vi "Teleop.vi"(10 "Match Info":T1={"Autonomous Elapsed Seconds"=0.0, "TeleOp Elapsed Seconds"=0.0, "Disabled Elapsed Seconds"=0.0, "Visited Autonomous"=FALSE, "Visited TeleOp"=FALSE, "Visited Disabled"=FALSE, "Autonomous Settings"={"Autonomous Style"=enum."Independent", "VI Refnum"=refnum}}, 11 "Call Context":T2) -> ()   [LabVIEW 2012]
doc: "This VI is called for each TeleOp packet received from the DS where the robot is not disabled. It is often used to read from the joysticks and update I/O or to update setpoints for timed control loops. It should complete and return within 20 milliseconds or it may miss DS packets."
uses:
  <vilib>/Rock Robotics/WPI/DriverStation/WPI_DriverStationDerivedRobotMode.ctl
  <vilib>/Rock Robotics/WPI/DriverStation/WPI_DriverStationMatch Info.ctl
  Robot Global Data.vi
  <vilib>/Rock Robotics/WPI/Solenoid/Deprecated/WPI_SolenoidSetBool.vi
  <vilib>/Rock Robotics/WPI/Joystick/WPI_JoystickGetSetRefNum.vi
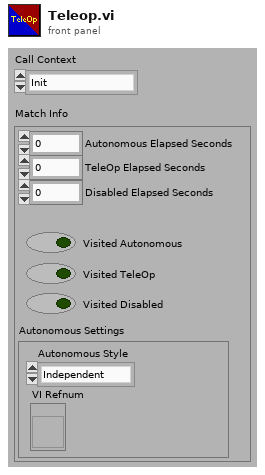
[diagram p1: front panel]
types:
  T1 = typedef "WPI_DriverStationMatch Info.ctl" = cluster{"Autonomous Elapsed Seconds":dbl, "TeleOp Elapsed Seconds":dbl, "Disabled Elapsed Seconds":dbl, "Visited Autonomous":bool, "Visited TeleOp":bool, "Visited Disabled":bool, "Autonomous Settings":cluster{"Autonomous Style":enum16{"Iterative", "Independent"}, "VI Refnum":refnum<vi>}}
  T2 = typedef "WPI_DriverStationDerivedRobotMode.ctl" = enum16{"Init", "Execute", "Stop"}
  T3 = typedef "WPI_DigitalInputDevRef.ctl" = cluster{"DevStatus":errorcluster, "DIO Channel":T4, "Digital Module":T5}
  T4 = typedef "FPGA_DIOChannel.ctl" = enum8{"DIO 1", "DIO 2", "DIO 3", "DIO 4", "DIO 5", "DIO 6", "DIO 7", "DIO 8", "DIO 9", "DIO 10", "DIO 11", "DIO 12", "DIO 13", "DIO 14", "Invalid"}
  T5 = typedef "FPGA_TypedefDigitalModule.ctl" = enum16{"Digital Module 1", "Digital Module 2"}
  T6 = typedef "WPI_SolenoidDevRef.ctl" = cluster{"DevStatus":errorcluster, "Solenoid Module":T7, "Forward Solenoid Channel":T8, "Reverse Solenoid Channel":T8}
  T7 = typedef "FPGA_TypedefSolenoidModule.ctl" = enum16{"Solenoid Module 1", "Solenoid Module 2"}
  T8 = typedef "WPI_SolenoidChannel.ctl" = enum8{"Solenoid 1", "Solenoid 2", "Solenoid 3", "Solenoid 4", "Solenoid 5", "Solenoid 6", "Solenoid 7", "Solenoid 8", "Invalid"}
  T9 = typedef "WPI_MotorControlDeviceRef.ctl" = cluster{"DeviceStatus":errorcluster, "Type":enum16{"PWM", "CAN"}, "PWM":cluster{"Digital Module":T5, "PWM Channel":T10, "DeadBand":T11}, "CAN":cluster{"Device Number":u8, "Control Mode":T12, "Semaphore":T13, "Max Vout":dbl}, "Invert":bool, "TransformRef":T14, "InvTransformRef":T14}
  T10 = typedef "FPGA_DIOPWMChannel.ctl" = enum8{"PWM 1", "PWM 2", "PWM 3", "PWM 4", "PWM 5", "PWM 6", "PWM 7", "PWM 8", "PWM 9", "PWM 10", "Invalid"}
  T11 = typedef "WPI_PWMDeadband.ctl" = cluster{"Name":string, "maxPositivePwm":i32, "minPositivePwm":i32, "centerPwm":i32, "maxNegativePwm":i32, "minNegativePwm":i32, "angularRange":u16}
  T12 = typedef "WPI_CANJaguar_ControlMode.ctl" = enum8{"Percent VBus", "Current", "Speed", "Position", "Voltage"}
  T13 = typedef "Semaphore RefNum" = refnum<k1>
  T14 = typedef "WPI_PWMTransform_ConPane.ctl" = refnum<vi>
  T15 = typedef "WPI_JoystickDevRef.ctl" = cluster{"Device":T16}
  T16 = typedef "WPI_JoystickDeviceEnum.ctl" = enum16{"USB 1", "USB 2", "USB 3", "USB 4", "Kinect 1", "Kinect 2"}
  T17 = typedef "WPI_JoystickButtonState.ctl" = cluster{"Button 1":bool, "Button 2":bool, "Button 3":bool, "Button 4":bool, "Button 5":bool, "Button 6":bool, "Button 7":bool, "Button 8":bool, "Button 9":bool, "Button 10":bool, "Button 11":bool, "Button 12":bool}
  T18 = cluster{"axis 1 (x)":dbl, "axis 2 (y)":dbl, "axis 3 (throttle)":dbl, "axis 4":dbl, "axis 5":dbl, "axis 6":dbl}
  T19 = typedef "WPI_RobotDriveDevRef.ctl" = cluster{"DevStatus":errorcluster, "Motors[]":T9[], "Square Inputs":bool, "Max Output":dbl, "Isochronous":bool}
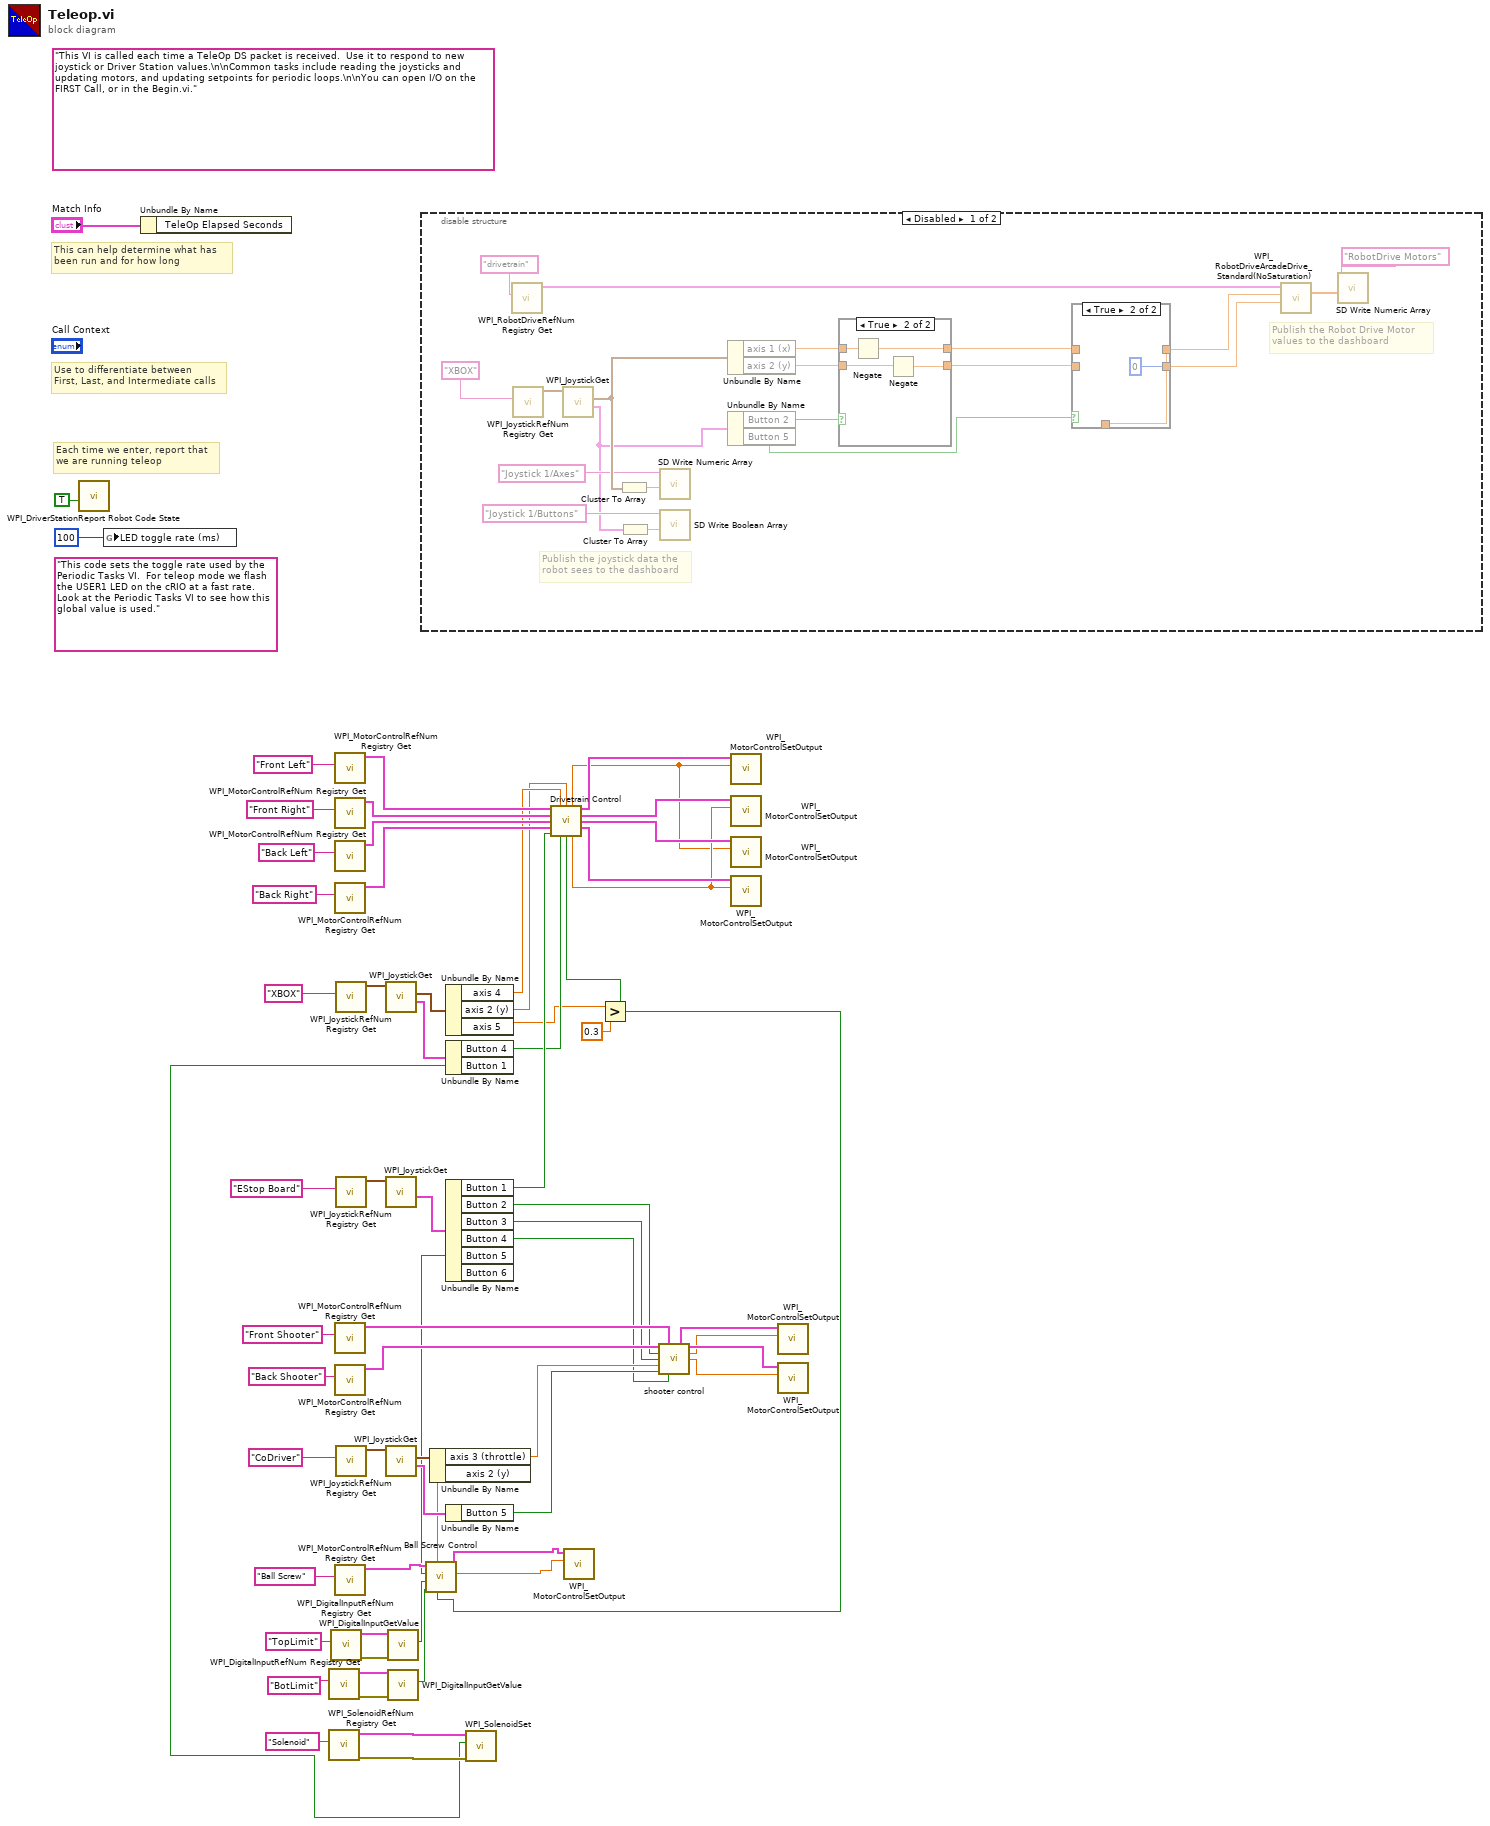
[diagram p0: block diagram]
diagram:
  (unwired) "This code sets the toggle rate used by the Periodic Tasks VI.  For teleop mode we flash the USER1 LED on the cRIO at a fast rate.  Look at the Periodic Tasks VI to see how this global value is used."
  (unwired) "This VI is called each time a TeleOp DS packet is received.  Use it to respond to new joystick or Driver Station values.\n\nCommon tasks include reading the joysticks and updating motors, and updating setpoints for periodic loops.\n\nYou can open I/O on the FIRST Call, or in the Begin.vi."
  # "Each time we enter, report that\nwe are running teleop"
  # "Use to differentiate between\nFirst, Last, and Intermediate calls"
  # "This can help determine what has\nbeen run and for how long"
  n1 = call <vilib>:"WPI_DriverStationReport Robot Code State.vi"("TeleOp"=TRUE ("Autonomous")) -> ()  [unwired: 10 in, 1 out]
  n2 = global write "Robot Global Data.vi" "LED toggle rate (ms)"(u32 100 ("LED ms toggle rate")) -> ()
  n3 = Unbundle By Name("Match Info") -> ()  [unwired: 1 out]
  n4 = call <vilib>:"WPI_DigitalInputRefNum Registry Get.vi"("refnum name"="BotLimit") -> ("error out"=w14:errorcluster, "DigitalInputDevRef"=w13:T3)  [unwired: 9 in]
  n5 = call <vilib>:"WPI_SolenoidRefNum Registry Get.vi"("refnum name"="Solenoid") -> ("error out"=w2:errorcluster, "SolenoidDevRef"=w3:T6)  [unwired: 9 in]
  n6 = call <vilib>:"WPI_DigitalInputRefNum Registry Get.vi"("refnum name"="TopLimit") -> ("error out"=w16:errorcluster, "DigitalInputDevRef"=w15:T3)  [unwired: 9 in]
  n7 = call <vilib>:"WPI_MotorControlRefNum Registry Get.vi"("refnum name"="Front Left") -> ("MotorControlDevRef"=w56:T9)  [unwired: 9 in, 1 out]
  n8 = call <vilib>:"WPI_MotorControlRefNum Registry Get.vi"("refnum name"="Front Right") -> ("MotorControlDevRef"=w55:T9)  [unwired: 9 in, 1 out]
  n9 = call <vilib>:"WPI_MotorControlRefNum Registry Get.vi"("refnum name"="Back Left") -> ("MotorControlDevRef"=w54:T9)  [unwired: 9 in, 1 out]
  n10 = call <vilib>:"WPI_MotorControlRefNum Registry Get.vi"("refnum name"="Back Right") -> ("MotorControlDevRef"=w53:T9)  [unwired: 9 in, 1 out]
  n11 = call <vilib>:"WPI_MotorControlRefNum Registry Get.vi"("refnum name"="Front Shooter") -> ("MotorControlDevRef"=w31:T9)  [unwired: 9 in, 1 out]
  n12 = call <vilib>:"WPI_MotorControlRefNum Registry Get.vi"("refnum name"="Back Shooter") -> ("MotorControlDevRef"=w32:T9)  [unwired: 9 in, 1 out]
  n13 = call <vilib>:"WPI_MotorControlRefNum Registry Get.vi"("refnum name"="Ball Screw") -> ("MotorControlDevRef"=w18:T9)  [unwired: 9 in, 1 out]
  n14 = call <vilib>:"WPI_JoystickRefNum Registry Get.vi"("refnum name"="XBOX") -> ("JoystickDevRef"=w51:T15)  [unwired: 1 in, 9 out]
  n15 = call <vilib>:"WPI_JoystickRefNum Registry Get.vi"("refnum name"="EStop Board") -> ("JoystickDevRef"=w41:T15)  [unwired: 1 in, 9 out]
  n16 = call <vilib>:"WPI_JoystickRefNum Registry Get.vi"("refnum name"="CoDriver") -> ("JoystickDevRef"=w45:T15)  [unwired: 1 in, 9 out]
  n17 = call <vilib>:"WPI_JoystickGet.vi"("JoystickDevRef"=w51) -> ("Buttons"=w47:T17, "Axes"=w50:T18)  [unwired: 1 in, 4 out]
  n18 = call <vilib>:"WPI_JoystickGet.vi"("JoystickDevRef"=w41) -> ("Buttons"=w40:T17)  [unwired: 1 in, 5 out]
  n19 = call <vilib>:"WPI_JoystickGet.vi"("JoystickDevRef"=w45) -> ("Buttons"=w43:T17, "Axes"=w44:T18)  [unwired: 1 in, 4 out]
  n20 = call <vilib>:"WPI_DigitalInputGetValue.vi"("error in (no error)"=w16, "DigitalInputDevRef"=w15) -> ("Value"=w12:bool)  [unwired: 7 in, 2 out]
  n21 = call <vilib>:"WPI_DigitalInputGetValue.vi"("error in (no error)"=w14, "DigitalInputDevRef"=w13) -> ("Value"=w11:bool)  [unwired: 7 in, 2 out]
  n22 = disable-structure shown="Disabled" {
    frame Disabled {
      # "Publish the Robot Drive Motor\nvalues to the dashboard"
      # "Publish the joystick data the\nrobot sees to the dashboard"
      n23 = call <vilib>:"WPI_RobotDriveRefNum Registry Get.vi"("refnum name"="drivetrain") -> ("RobotDriveDevRef"=w86:T19)  [unwired: 1 in, 9 out]
      n24 = call <vilib>:"WPI_JoystickRefNum Registry Get.vi"("refnum name"="XBOX") -> ("JoystickDevRef"=w84:T15)  [unwired: 1 in, 9 out]
      n25 = call <vilib>:"WPI_JoystickGet.vi"("JoystickDevRef"=w84) -> ("Buttons"=w76:T17, "Axes"=w81:T18)  [unwired: 1 in, 4 out]
      n26 = Cluster To Array(cluster=w81) -> (array=w80:dbl[])
      n27 = Cluster To Array(cluster=w76) -> (array=w83:bool[])
      n28 = call <vilib>:"SD Write Numeric Array.vi"("Numeric Array"=w80, "Name"="Joystick 1/Axes") -> ()  [unwired: 8 in, 2 out]
      n29 = call <vilib>:"SD Write Boolean Array.vi"("Boolean Array"=w83, "Name"="Joystick 1/Buttons") -> ()  [unwired: 8 in, 2 out]
      n30 = Unbundle By Name(w81) -> ("axis 1 (x)"=w74:dbl, "axis 2 (y)"=w73:dbl)
      n31 = Unbundle By Name(w76) -> ("Button 2"=w75:bool, "Button 5"=w72:bool)
      n32 = case shown="True" w75 {
        tunnel: [w93 w94] -> w70
        tunnel: w74 -> [w93 w97]
        tunnel: [w92 w95] -> w68
        tunnel: w73 -> [w92 w96]
        frame False {
        }
        frame True {
          n33 = Negate(x=w97) -> (-x=w94:dbl)
          n34 = Negate(x=w96) -> (-x=w95:dbl)
        }
      }
      n35 = case shown="True" w72 {
        tunnel: [w89 w90] -> w71
        tunnel: w70 -> [w89 _]
        tunnel: [w88 0] -> w69
        tunnel: w68 -> [w88 _]
        tunnel: [_ w90] -> w67
        frame False {
        }
        frame True {
        }
      }
      n36 = call <vilib>:"WPI_RobotDriveArcadeDrive_Standard(NoSaturation).vi"("Y axis value"=w69, "X axis value"=w71, "RobotDriveDevRef"=w86) -> ("Motor Values"=w77:dbl[])  [unwired: 1 in, 7 out]
      n37 = call <vilib>:"SD Write Numeric Array.vi"("Numeric Array"=w77, "Name"="RobotDrive Motors") -> ()  [unwired: 8 in, 2 out]
    }
    frame Enabled {
    }
  }
  n38 = Unbundle By Name(w44) -> ("axis 3 (throttle)"=w25:dbl, "axis 2 (y)"=w10:dbl)
  n39 = Unbundle By Name(w50) -> ("axis 4"=w49:dbl, "axis 2 (y)"=w48:dbl, "axis 5"=w8:dbl)
  n40 = Unbundle By Name(w47) -> ("Button 4"=w21:bool, "Button 1"=w1:bool)
  n41 = Unbundle By Name(w40) -> ("Button 1"=w33:bool, "Button 2"=w24:bool, "Button 3"=w23:bool, "Button 4"=w22:bool, "Button 5"=w17:bool)  [unwired: 1 out]
  n42 = Unbundle By Name(w43) -> ("Button 5"=w26:bool)
  n43 = call-poly <vilib>:"WPI_SolenoidSet.vi"("error in (no error)"=w2, "Value"=w1, "SolenoidDevRef"=w3) -> ()  [unwired: 7 in, 2 out]
  n44 = Greater?(x=w8, y=0.3) -> (0:w7:bool)
  n45 = call "Ball Screw Control.vi"("Target"=w7, "Axis"=w10, "BotLimit"=w11, "TopLimit"=w12, "Closed Loop On/Off"=w17, "Ball Screw DevRef In"=w18) -> ("Motor Output"=w5:dbl, "Ball Screw DevRef Out"=w6:T9)  [unwired: 4 in]
  n46 = call "Drivetrain Control.vi"("Back Left DevRef In"=w56, "X Axis"=w49, "Y Axis"=w48, "Back Right DevRef In"=w55, "Front Left DevRef In"=w54, "Front Right DevRef In"=w53, "Closed Loop On/Off"=w33, "Drivetrain Reverse Button"=w21, "Trigger"=w7) -> ("Left Motor Value"=w34:dbl, "Back Left DevRef Out"=w39:T9, "Back Right DevRef Out"=w38:T9, "Front Left DevRef Out"=w37:T9, "Front Right DevRef Out"=w36:T9, "Right Motor Value"=w35:dbl)  [unwired: 1 in]
  n47 = call <vilib>:"WPI_MotorControlSetOutput.vi"("Output"=w5, "MotorControlDevRef"=w6) -> ()  [unwired: 7 in, 3 out]
  n48 = call "shooter control.vi"("Back Shooter DevRef In"=w32, "Front Shooter DevRef In"=w31, "Closed Loop On/Off"=w24, "Power On/Off"=w23, "Joystick Throttle"=w25, "Target Button"=w26, "shooter control.viPyramidButton"=w22) -> ("Front Shooter DevRef Out"=w30:T9, "Back Shooter DevRef Out"=w29:T9, "FrontShooterOut"=w28:dbl, "BackShooterOut"=w27:dbl)  [unwired: 5 in]
  n49 = call <vilib>:"WPI_MotorControlSetOutput.vi"("Output"=w34, "MotorControlDevRef"=w39) -> ()  [unwired: 7 in, 3 out]
  n50 = call <vilib>:"WPI_MotorControlSetOutput.vi"("Output"=w35, "MotorControlDevRef"=w38) -> ()  [unwired: 7 in, 3 out]
  n51 = call <vilib>:"WPI_MotorControlSetOutput.vi"("Output"=w34, "MotorControlDevRef"=w37) -> ()  [unwired: 7 in, 3 out]
  n52 = call <vilib>:"WPI_MotorControlSetOutput.vi"("Output"=w35, "MotorControlDevRef"=w36) -> ()  [unwired: 7 in, 3 out]
  n53 = call <vilib>:"WPI_MotorControlSetOutput.vi"("Output"=w28, "MotorControlDevRef"=w30) -> ()  [unwired: 7 in, 3 out]
  n54 = call <vilib>:"WPI_MotorControlSetOutput.vi"("Output"=w27, "MotorControlDevRef"=w29) -> ()  [unwired: 7 in, 3 out]
